vi "writeToClient.vi"(8 "error in (no error)":errorcluster, 10 "packet":string, 11 "tcpServerCmd in":refnum<class "TcpServerCmd.lvclass">) -> (0 "error out":errorcluster, 3 "tcpServerCmd out":refnum<class "TcpServerCmd.lvclass">)   [LabVIEW 2018, in "TcpServerCmd.lvclass"]
doc: "Write packet to the TCP Client."
uses:
  TcpServerCmd.lvclass
  home/pcortes/github/ts_labview_tcp_json/src/TcpServerBase/TcpServerBase.lvclass
  TcpServerBase/TcpServerBase.lvclass/TcpServerBase.ctl
  TcpServerBase/TcpServerBase.lvclass
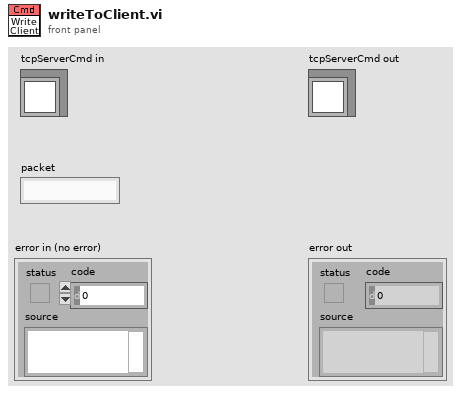
[diagram p1: front panel]
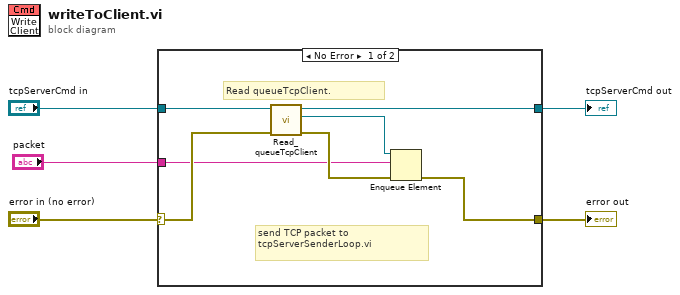
[diagram p0: block diagram]
diagram:
  n1 = case shown="No Error" "error in (no error)" {
    selector: "error in (no error)" -> [w8 w14]
    tunnel: [w7 w14] -> w4
    tunnel: [w9 w13] -> w2
    tunnel: "tcpServerCmd in" -> [w10 w13]
    tunnel: "packet" -> [w6 _]
    frame No Error {
      # "send TCP packet to\ntcpServerSenderLoop.vi"
      # "Read queueTcpClient."
      n2 = call "Read_queueTcpClient.vi"("error in (no error)"=w8, "TcpServerBase in"=w10) -> ("error out"=w11:errorcluster, "queueTcpClient"=w12:refnum<queue>, "TcpServerBase out"=w9:refnum<class "TcpServerCmd.lvclass">)  [unwired: 7 in]
      n3 = Enqueue Element(queue=w12, element=w6, error in (no error)=w11) -> (error out=w7:errorcluster)  [unwired: 1 in, 2 out]
    }
    frame Error {
    }
  }
  "error out" <- w4
  "tcpServerCmd out" <- w2
